vi "Process indexed triangle.vi"(1 "Triangle in (indexed)":T1={"V0"=[], "V1"=[], "V2"=[], "n^"=[], "i0"=-1, "i1"=-1, "i2"=-1}) -> (0 "Triangle out (indexed)":T1={"V0"=[], "V1"=[], "V2"=[], "n^"=[], "i0"=-1, "i1"=-1, "i2"=-1})   [LabVIEW 2014]
doc: "This VI must be run after any alteration to the triangles geometry involving scaling and rotation.\nThere is no need to run this VI after applying a translation."
uses:
  Typedefs/Triangle, indexed.ctl
  Subroutines/Cross product 3D.vi
  Subroutines/Unit vector.vi
  Subroutines/Dot product.vi
panel:
  # "PN 29/03/2015"
  # "Vertices"
  # "Indices"
  # "Unit normal"
  # "Vertices"
  # "Indices"
  # "Unit normal"
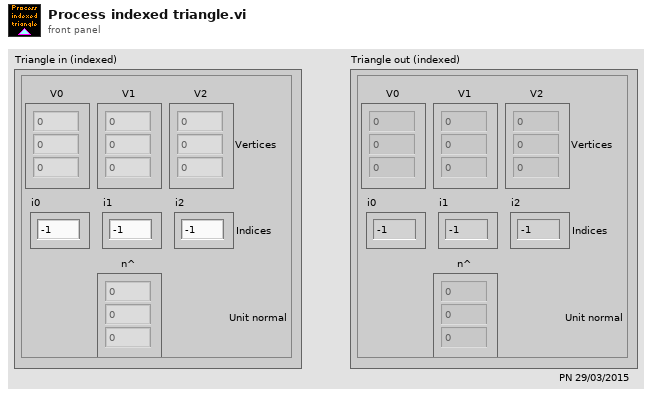
[diagram p1: front panel]
types:
  T1 = typedef "Triangle, indexed.ctl" = cluster{"V0":sgl[], "V1":sgl[], "V2":sgl[], "n^":sgl[], "i0":i32, "i1":i32, "i2":i32}
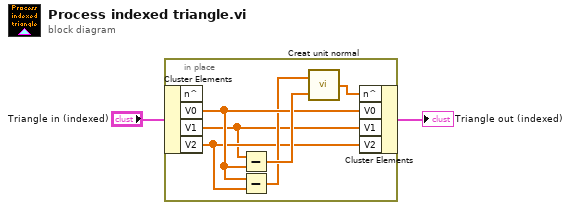
[diagram p0: block diagram]
diagram:
  n1 = in-place {
    n2 = in-place-cluster #1("Triangle in (indexed)") -> ("V0"=w6:sgl[], "V1"=w3:sgl[], "V2"=w4:sgl[])  [unwired: 1 out]
    n3 = Subtract(x=w3, y=w6) -> (x-y=w7:sgl[])
    n4 = Subtract(x=w6, y=w4) -> (x-y=w5:sgl[])
    n5 = call "Creat unit normal.vi"("E2"=w7, "E1"=w5) -> ("n^ = (E1 x E2) / ||E1 x E2||"=w8:sgl[])
    n6 = in-place-cluster #1("n^"=w8, "V0"=w6, "V1"=w3, "V2"=w4) -> (→"Triangle out (indexed)":T1)
  }
